vi "LVClasse_Phase ctor from ModalCoef.vi"(0 "Phase (const)":refnum<class "Phase.lvclass">, 5 "ModalCoef":refnum<class "ModalCoef.lvclass">, 7 "Filter":u8[](array[numeric]), 11 "error in (no error)":errorcluster) -> (4 "Phase (new)":refnum<class "Phase.lvclass">, 6 "ModalCoef (dup)":refnum<class "ModalCoef.lvclass">, 15 "error out":errorcluster)   [LabVIEW 2020, in "Phase.lvclass"]
doc: "Phase constructor from ModalCoef.\n\n<B>PhaseIn</B> : Constant Pointer to Phase object. Phase sampling sizes and steps are set from\n ModalCoef object (Pupil object sizes).\n<B>PhaseOut</B> : Constant Pointer to Phase object. Phase sampling sizes and steps are set from\n ModalCoef object (Pupil object sizes).\n<B>ModalCoef</B> : ModalCoef object.\n<B>filter</B> : Array of aberrations to filter."
uses:
  Phase.lvclass
  ModalCoef.lvclass
  Handle creation.ctl
  Phase.lvclass/Phase.ctl
  LVClass_ModalCoef Read ModalCoef.vi
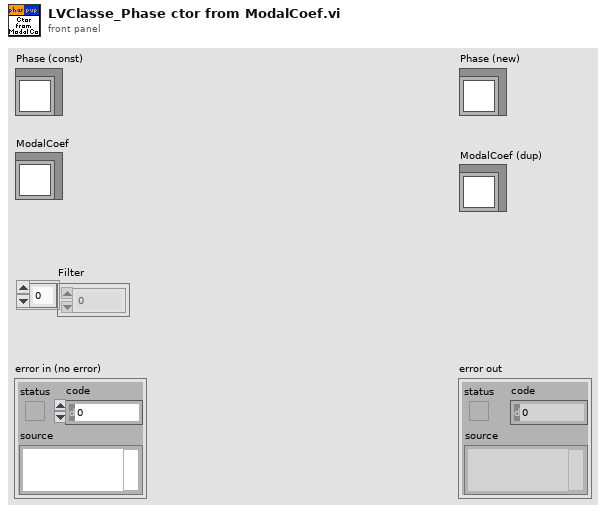
[diagram p1: front panel]
types:
  T1 = typedef "Handle creation.ctl" = enum16{"By ctor", "By write function"}
  T2 = typedef "ClassID.ctl" = i64
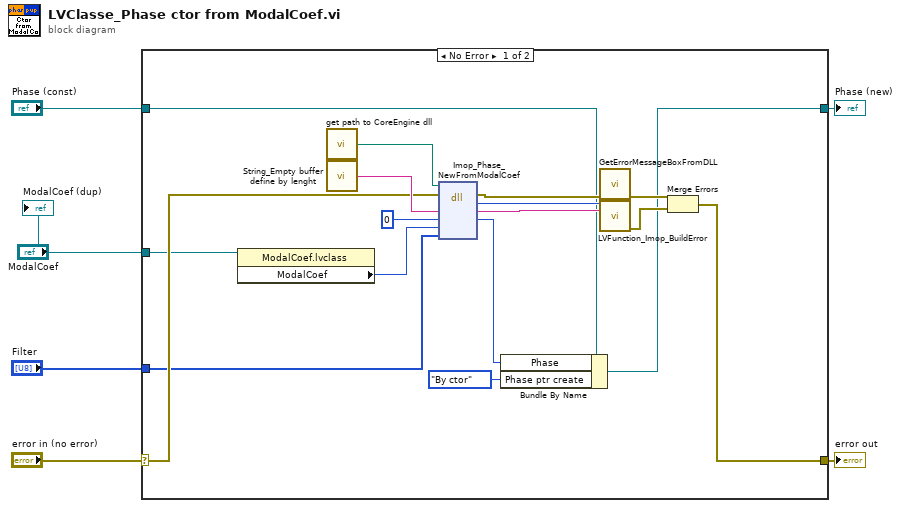
[diagram p0: block diagram]
diagram:
  n1 = case shown="No Error" "error in (no error)" {
    selector: "error in (no error)" -> [w16 w25]
    tunnel: [w15 w25] -> w5
    tunnel: [w8 w24] -> w3
    tunnel: "Phase (const)" -> [w9 w24]
    tunnel: "ModalCoef" -> [w14 _]
    tunnel: "Filter" -> [w12 _]
    frame No Error {
      n2 = property class="ModalCoef.lvclass"(reference=w14) -> ("ModalCoef"=w13:T2)  [unwired: 1 in, 2 out]
      n3 = call "get path to CoreEngine dll.vi"() -> ("path to wavekit library"=w20:path)  [unwired: 14 in, 1 out]
      n4 = call "String_Empty buffer define by lenght.vi"() -> ("Empty buffer"=w21:string)  [unwired: 1 in]
      n5 = dll-call lib="D:/FLE/0.Code/CoreEngine4_Suite/LV2011_interface/DLLs/c_interface_vc100.dll" fn="Imop_Phase_NewFromModalCoef"(path in=w20, error in=w16, "message"=w21, "Phase"=0, "ModalCoef"=w13, "Filter"=w12) -> (error out=w19:errorcluster, "return type"=w23:i32, "message"=w22:string, "Phase"=w11:i64)  [unwired: 3 in, 1 out]
      n6 = Bundle By Name(cluster=w9, "Phase"=w11, "Phase ptr create"=Handle_creation."By ctor") -> (w8:refnum<class "Phase.lvclass">)
      n7 = call "GetErrorMessageBoxFromDLL.vi"("error IN"=w19) -> ("error OUT"=w18:errorcluster)  [unwired: 10 in]
      n8 = call "LVFunction_Imop_BuildError.vi"("code"=w23, "String to Prepend to source (\"\")"=w22) -> ("error out"=w17:errorcluster)  [unwired: 13 in]
      n9 = Merge Errors(w18, w17) -> (w15:errorcluster)
    }
    frame Error {
    }
  }
  "error out" <- w5
  "Phase (new)" <- w3
  "ModalCoef (dup)" <- "ModalCoef"
